vi "Untitled 2 (SubVI).vi"(11 "Numeric in":dbl) -> (3 "Numeric out":dbl)   [LabVIEW 2019]
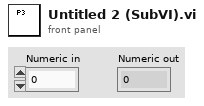
[diagram p1: front panel]
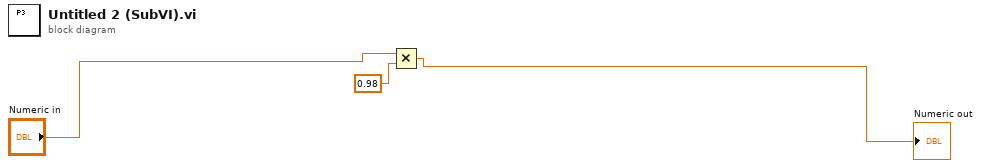
[diagram p0: block diagram]
diagram:
  n1 = Multiply(x="Numeric in", y=0.98) -> (x*y=→"Numeric out":dbl)
